vi "Get Next Generation Outputs.vi"(8 "error in":errorcluster, 10 "generation in":u32, 11 "cells in":bool[][](array[boolean])) -> (0 "error out":errorcluster, 1 "game of life":T1, 2 "generation out":u32, 3 "cells out":bool[][](array[boolean]), 4 "stop generation?":bool)   [LabVIEW 2021, in "Game of Life.lvlib"]
doc: "This VI generates the next generation of living cells by applying the game logic and convets them to XY coordinates of the game of life board."
uses:
  Game of Life.lvlib
  Game of Life Cluster.ctl
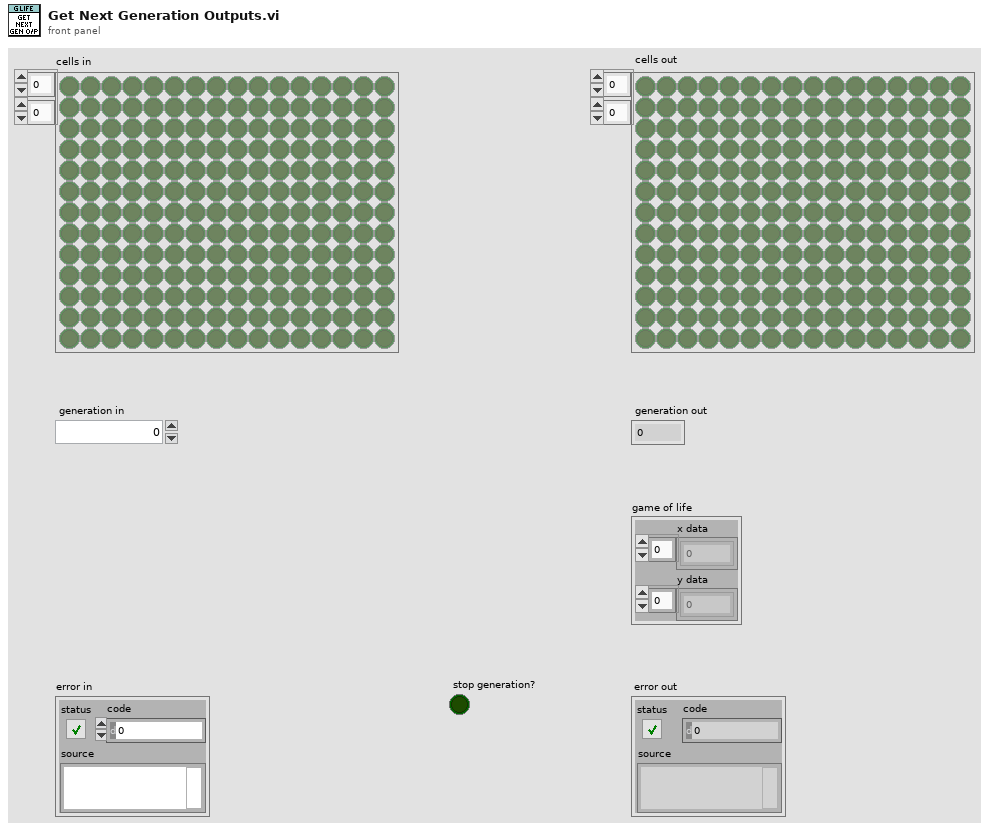
[diagram p1: front panel]
types:
  T1 = typedef "Game of Life.lvlib/Game of Life Cluster.ctl" = cluster{"x data":dbl[], "y data":dbl[]}
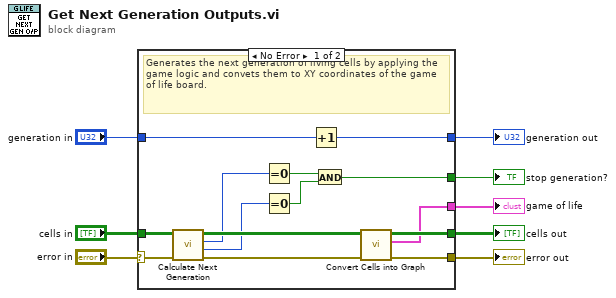
[diagram p0: block diagram]
diagram:
  n1 = case shown="No Error" "error in" {
    selector: "error in" -> [w22 w24]
    tunnel: "cells in" -> [w21 w23]
    tunnel: [w18 _] -> w4
    tunnel: "generation in" -> [w17 w25]
    tunnel: [w14 w24] -> w3
    tunnel: [w16 w25] -> w5
    tunnel: [w12 w23] -> w2
    tunnel: [w11 _] -> w1
    frame No Error {
      # "Generates the next generation of living cells by applying the game logic and convets them to XY coordinates of the game of life board."
      n2 = call "Calculate Next Generation.vi"("error in"=w22, "cells in"=w21) -> ("error out"=w15:errorcluster, "deaths"=w9:i32, "births"=w10:i32, "cells out"=w13:bool[][])  [unwired: 6 in]
      n3 = Equal To 0?(x=w10) -> (x = 0?=w19:bool)
      n4 = Equal To 0?(x=w9) -> (x = 0?=w20:bool)
      n5 = Increment(x=w17) -> (x+1=w16:u32)
      n6 = And(x=w19, y=w20) -> (x .and. y?=w18:bool)
      n7 = call "Convert Cells into Graph.vi"("error in"=w15, "cells in"=w13) -> ("error out"=w14:errorcluster, "game of life"=w11:T1, "cells out"=w12:bool[][])  [unwired: 7 in]
    }
    frame Error {
    }
  }
  "generation out" <- w5
  "stop generation?" <- w4
  "cells out" <- w2
  "error out" <- w3
  "game of life" <- w1
